vi "Parse HTTP Header Line.vi"(8 "error in (no error)":errorcluster, 10 "HTTP Header Line":string, 11 "WebSocket Server in":refnum<class "WebSocket Server.lvclass">) -> (0 "error out":errorcluster, 3 "WebSocket Server out":refnum<class "WebSocket Server.lvclass">)   [LabVIEW 2021, in "WebSockets.lvlib" / "WebSocket Server.lvclass"]
doc: "Parses the first row of the HTTP request to determine the method/URI/protocol.\nWebSockets 2.0.1.40\nSam Sharp - MediaMongrels Ltd\nCopyright (c) 2019, MediaMongrels Ltd"
uses:
  WebSocket Server.lvclass
  WebSocket Server.lvclass/WebSocket Server.ctl
panel:
  out "Protocol":string
  out "Method":string
  out "Request URI":string
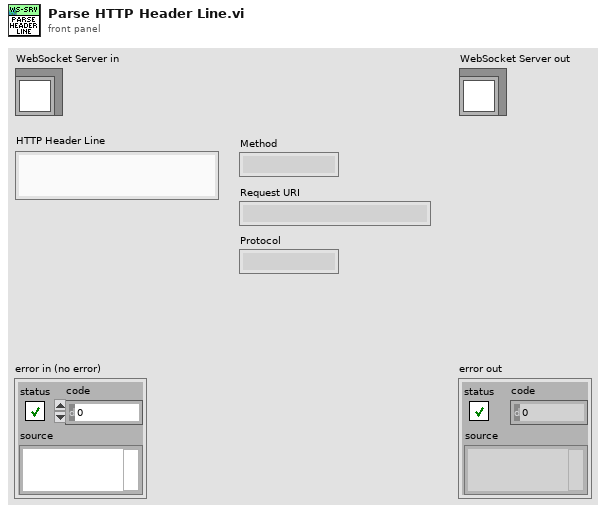
[diagram p1: front panel]
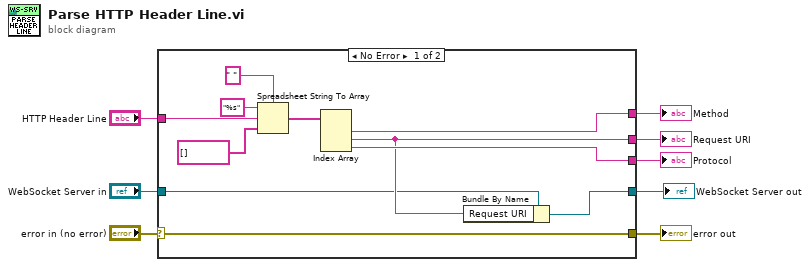
[diagram p0: block diagram]
diagram:
  n1 = case shown="No Error" "error in (no error)" {
    selector: "error in (no error)" -> [w9 w21]
    tunnel: "HTTP Header Line" -> [w16 _]
    tunnel: [w12 _] -> w8
    tunnel: [w14 _] -> w7
    tunnel: [w13 _] -> w6
    tunnel: [w9 w21] -> w4
    tunnel: [w10 w20] -> w2
    tunnel: "WebSocket Server in" -> [w11 w20]
    frame No Error {
      n2 = Spreadsheet String To Array(delimiter (Tab)=" ", format string="%s", spreadsheet string=w16, array type (2D Dbl)=string[] []) -> (array=w18:string[])
      n3 = Index Array(array=w18) -> (element #1=w14:string, element #2=w12:string, element #3=w13:string)  [unwired: 3 in]
      n4 = Bundle By Name(cluster=w11, "Request URI"=w12) -> (w10:refnum<class "WebSocket Server.lvclass">)
    }
    frame Error {
    }
  }
  "error out" <- w4
  "WebSocket Server out" <- w2
  "Request URI" <- w8
  "Method" <- w7
  "Protocol" <- w6
